vi "SLSC Get SLSC Chassis Address in Host.vi"(8 "error in (no error)":errorcluster, 11 "Node Ptr":T1 format="%.0x") -> (0 "error out":errorcluster, 1 "ChassisIDType":i32(ring) items=["ChassisName", "HostnameIPAddress"], 2 "IP Address":string, 3 "Node Ptr":T1 format="%.0x", 4 "Password":string, 5 "Username":string)   [LabVIEW 2017, in "SLSC CD System Explorer.lvlib"]
uses:
  SLSC CD System Explorer.lvlib
  <vilib>/NI Veristand/Custom Device API/Custom Device Item Ref.ctl
  NationalInstruments.VeriStand.SystemDefinitionAPI
  <vilib>/NI Veristand/Custom Device API/Custom Device API.lvlib
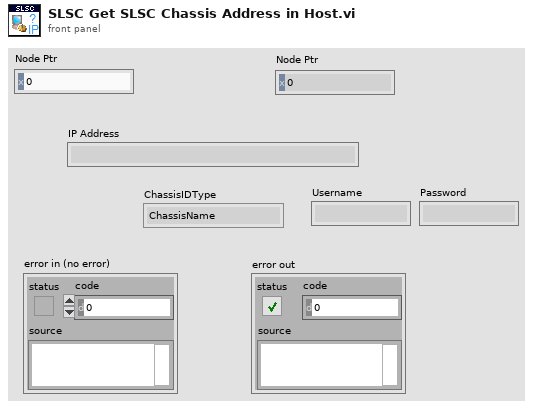
[diagram p1: front panel]
types:
  T1 = typedef "Custom Device API.lvlib/Custom Device Item Ref.ctl" = u64
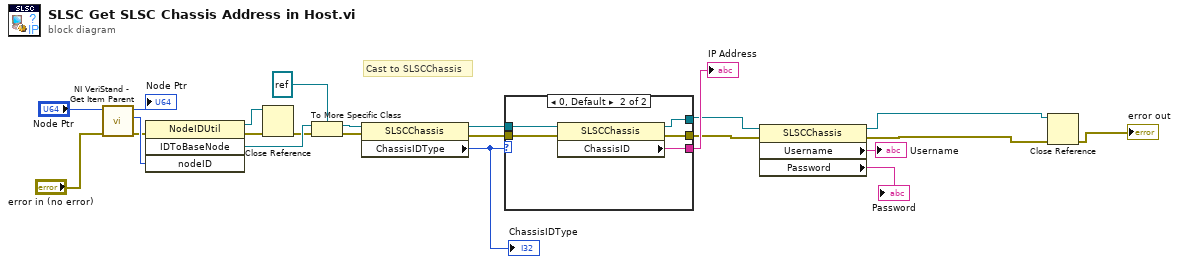
[diagram p0: block diagram]
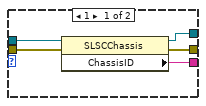
[diagram p2: hidden frame]
diagram:
  # "Cast to SLSCChassis"
  n1 = call <vilib>:"NI VeriStand - Get Item Parent.vi"("error in (no error)"="error in (no error)", "Item Ref in"="Node Ptr") -> ("error out"=w21:errorcluster, "Parent Ref"=w23:T1, "Item Ref out"=→"Node Ptr":T1)  [unwired: 6 in, 1 out]
  n2 = invoke class="NodeIDUtil" method="IDToBaseNode"(error in=w21, "nodeID"=w23) -> (reference out=w15:refnum<k24>, error out=w16:errorcluster, "IDToBaseNode"=w18:refnum<k24>)  [unwired: 2 in, 1 out]
  n3 = Close Reference(reference=w15, error in (no error)=w16) -> (error out=w17:errorcluster)
  n4 = To More Specific Class(target class=refnum<k24> refnum, reference=w18, error in=w17) -> (specific class reference=w12:refnum<k24>, error out=w11:errorcluster)
  n5 = property class="SLSCChassis"(reference=w12, error in=w11) -> (reference out=w10:refnum<k24>, error out=w9:errorcluster, "ChassisIDType"=w8:i32)
  "ChassisIDType" <- w8
  n6 = case shown="0, Default" w8 {
    tunnel: [w28 w33] -> w20
    tunnel: w10 -> [w27 w32]
    tunnel: w9 -> [w26 w31]
    tunnel: [w25 w30] -> w6
    tunnel: [w24 w29] -> w5
    frame 1 {
      n7 = property class="SLSCChassis"(reference=w27, error in=w26) -> (reference out=w25:refnum<k24>, error out=w24:errorcluster, "ChassisID"=w28:string)
    }
    frame 0, Default {
      n8 = property class="SLSCChassis"(reference=w32, error in=w31) -> (reference out=w30:refnum<k24>, error out=w29:errorcluster, "ChassisID"=w33:string)
    }
  }
  "IP Address" <- w20
  n9 = property class="SLSCChassis"(reference=w6, error in=w5) -> (reference out=w4:refnum<k24>, error out=w3:errorcluster, "Username"=→"Username":string, "Password"=→"Password":string)
  n10 = Close Reference(reference=w4, error in (no error)=w3) -> (error out=→"error out":errorcluster)
